vi "readTPDO.vi"(8 "error in (no error)":errorcluster, 10 "TPDO object in":refnum<k20>, 11 "MotorController in":refnum<class "MotorController.lvclass">) -> (0 "error out":errorcluster, 1 "TPDO data":u8[](array[numeric]), 2 "TPDO object out":refnum<k20>, 3 "MotorController out":refnum<class "MotorController.lvclass">, 5 "new data?":bool)   [LabVIEW 2017, in "MotorController.lvclass"]
uses:
  MotorController.lvclass
  MotorController.lvclass/MotorController.ctl
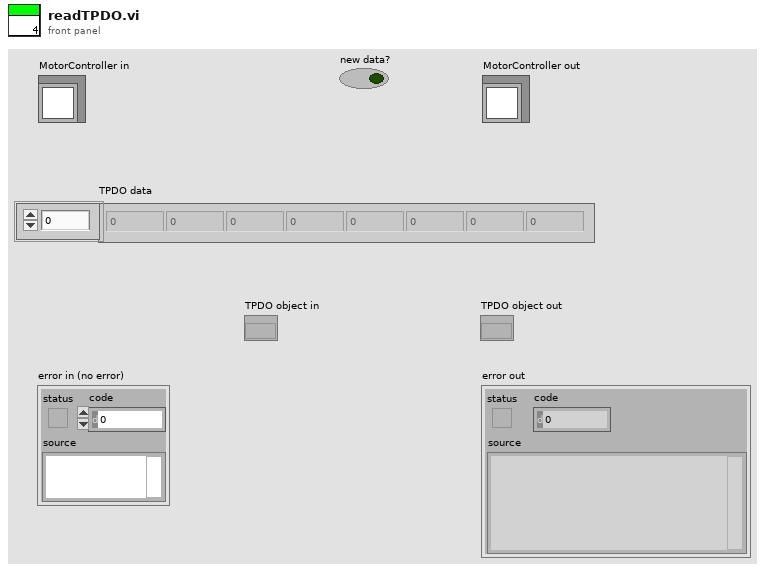
[diagram p1: front panel]
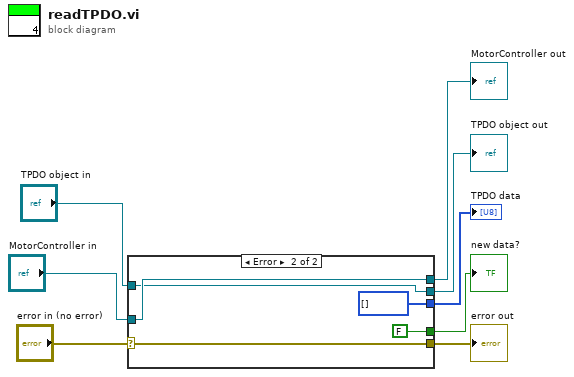
[diagram p0: block diagram]
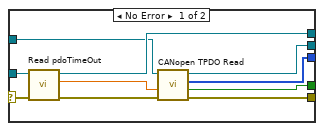
[diagram p2: hidden frame]
diagram:
  n1 = case shown="Error" "error in (no error)" {
    selector: "error in (no error)" -> [w12 w23]
    tunnel: [w9 w23] -> w7
    tunnel: [w16 w22] -> w5
    tunnel: "MotorController in" -> [w13 w22]
    tunnel: [w15 u8[] [] ("data")] -> w4
    tunnel: [w14 FALSE ("new data?")] -> w3
    tunnel: "TPDO object in" -> [w11 w19]
    tunnel: [w10 w19] -> w1
    frame No Error {
      n2 = call "Read pdoTimeOut.vi"("error in (no error)"=w12, "MotorController in"=w13) -> ("error out"=w17:errorcluster, "pdoTimeOut"=w18:dbl, "MotorController out"=w16:refnum<class "MotorController.lvclass">)  [unwired: 7 in]
      n3 = call <vilib>:"CANopen TPDO Read.vi"("error in (no error)"=w17, "timeout (0s)"=w18, "TPDO object in"=w11) -> ("error out"=w9:errorcluster, "new data?"=w14:bool, "data"=w15:u8[], "TPDO object out"=w10:refnum<k20>)  [unwired: 4 in, 1 out]
    }
    frame Error {
    }
  }
  "error out" <- w7
  "MotorController out" <- w5
  "TPDO data" <- w4
  "new data?" <- w3
  "TPDO object out" <- w1
